vi "ReadTemplate.vi"(8 "error in":errorcluster, 11 "ObjIn":refnum<class>) -> (0 "error out":errorcluster, 2 "PropOut":bool=TRUE, 3 "ObjOut":refnum<class>)   [LabVIEW 2013]
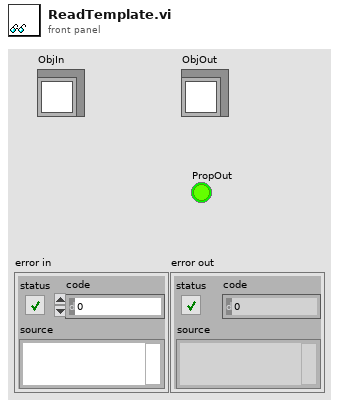
[diagram p1: front panel]
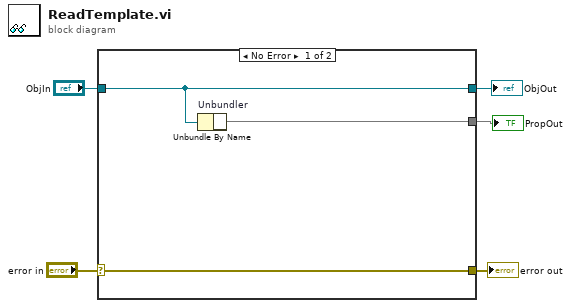
[diagram p0: block diagram]
diagram:
  n1 = case shown="No Error" "error in" {
    selector: "error in" -> [w8 w10]
    tunnel: "ObjIn" -> [w7 w9]
    tunnel: [w7 w9] -> w4
    tunnel: [w8 w10] -> w2
    tunnel: [w6 _] -> w1
    frame No Error {
      n2 = Unbundle By Name "Unbundler"(w7) -> (w6)
    }
    frame Error {
    }
  }
  "ObjOut" <- w4
  "error out" <- w2
  "PropOut" <- w1
